vi "Command2Angel.vi"(10 "DataIn":u8[](array[numeric])) -> (2 "AngelOut":dbl)   [LabVIEW 2013]
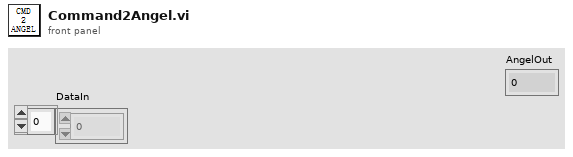
[diagram p1: front panel]
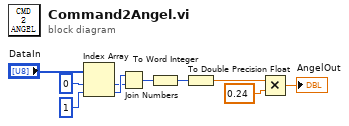
[diagram p0: block diagram]
diagram:
  n1 = Index Array(array="DataIn", index #1=0 ("index"), index #2=1 ("index")) -> (element #1=w6:u8, element #2=w7:u8)
  n2 = Join Numbers(hi=w7, lo=w6) -> ((hi.lo)=w5:u16)
  n3 = To Word Integer(number=w5) -> (16bit integer=w1:i16)
  n4 = To Double Precision Float(number=w1) -> (double precision float=w4:dbl)
  n5 = Multiply(x=w4, y=0.24) -> (x*y=→"AngelOut":dbl)
